vi "HFRR ADV v09.vi"() -> ()   [LabVIEW 2025] (continued)
        n1021 = call-poly "VISA Configure Serial Port"("VISA resource name"=refnum<visa-resource-name> "ASRL1::INSTR" ("COM PORT"), "timeout (10sec)"=u32 10, "baud rate (9600)"=u32 57600, "data bits (8)"=u16 8, "stop bits (10: 1 bit)"=w1236) -> ("VISA resource name out"=w1222:refnum<visa-resource-name>, "error out"=w1231:errorcluster)  [unwired: 9 in]
        n1022 = VISA Read(VISA resource name=w1222, byte count=u32 2 ("byte count (0)")) -> (read buffer=w1230:string)  [unwired: 1 in, 3 out]
        n1023 = String Subset(string=w1230, offset (0)=0, length (rest)=2 ("length (rest)")) -> (substring=w1229:string)
        n1024 = Match Pattern(string=w1229, regular expression="<>") -> (offset past match=w1226:i32)  [unwired: 1 in, 3 out]
        n1025 = Greater Or Equal?(x=w1226, y=0) -> (x >= y?=w1221:bool)
        n1026 = case shown="True" w1221 {
          tunnel: w1222 -> [_ w1240]
          tunnel: w1231 -> [_ w1239]
          frame False {
          }
          frame True {
            n1027 = VISA Read(VISA resource name=w1240, byte count=u32 32 ("byte count (0)"), error in (no error)=w1239) -> (read buffer=w1238:string)  [unwired: 3 out]
            n1028 = String Subset(string=w1238, offset (0)=0, length (rest)=8 ("length (rest)")) -> (substring=w1242:string)
            n1029 = String Subset(string=w1238, offset (0)=8, length (rest)=8 ("length (rest)")) -> (substring=w1243:string)
            n1030 = Decimal String To Number(string=w1243) -> (number=w1250:i32)  [unwired: 2 in, 1 out]
            n1031 = Decimal String To Number(string=w1242) -> (number=w1246:i32)  [unwired: 2 in, 1 out]
            n1032 = Divide(x=w1250, y=10000) -> ()  [unwired: 1 out]
            n1033 = Divide(x=w1246, y=1000000) -> ()  [unwired: 1 out]
          }
        }
        n1034 = local read "Quit"() -> (w1219:bool)
      }
    }
    frame Enabled {
    }
  }
  n1035 = local write "Err Count"(0 ("Err Count")) -> ()
  n1036 = local write "FRICVALZ"(0.0 ("FRICVALZ")) -> ()
  n1037 = Tick Count (ms)() -> (millisecond timer value=w44:u32)
  n1038 = while {
    shift-right: [w1269] -> w48
    shift-left: _ -> [w1258]
    shift-right: [w1268] -> w47
    shift-left: errorcluster {"status"=TRUE, "code"=0, "source"="Init"} ("error IO") -> [w1260]
    shift-right: [w1266] -> _
    shift-left: w44 -> [w1267]
    tunnel: [w1252] -> w35
    tunnel: [w1265] -> _
    i -> [w1265]
    stop <- w1252 stop-if-true
    n1039 = local read "Com Port 1"() -> (w1259:refnum<visa-resource-name>)
    n1040 = local read "Port 1a"() -> (w1261:bool)
    n1041 = local read "Port 3"() -> (w1262:bool)
    n1042 = Not Equal?(x=w1259, y=w1258) -> (x != y?=w1257:bool)
    n1043 = Or(x=w1262, y=w1261) -> (x .or. y?=w1264:bool)
    n1044 = Unbundle(w1260) -> ("status"=→"Port 3":bool)  [unwired: 2 out]
    n1045 = flat-sequence {
      tunnel: [w1272] -> w1256
      tunnel: w1260 -> [w1272]
      frame #0 {
        n1046 = Wait (ms)(milliseconds to wait=u32 200) -> ()  [unwired: 1 out]
      }
    }
    n1047 = case shown="False" w1264 {
      frame False {
        w1274 = FALSE ("Visible")
        n1048 = property on="Port 1a" class="Bool (strict)"("Visible"=w1274) -> ()  [unwired: 2 in, 2 out]
        n1049 = property on="Port 3" class="Bool (strict)"("Visible"=w1274) -> ()  [unwired: 2 in, 2 out]
      }
      frame True {
        w1275 = TRUE ("Visible")
        n1050 = property on="Port 1a" class="Bool (strict)"("Visible"=w1275) -> ()  [unwired: 2 in, 2 out]
        n1051 = property on="Port 3" class="Bool (strict)"("Visible"=w1275) -> ()  [unwired: 2 in, 2 out]
      }
    }
    n1052 = local read "Re-Initialise"() -> (w1253:bool)
    n1053 = Or(x=w1257, y=w1253) -> (x .or. y?=w1254:bool)
    n1054 = case shown="True" w1254 {
      tunnel: [w1270 errorcluster {"status"=TRUE, "code"=0, "source"="Init"} ("error out")] -> w1255
      tunnel: w1256 -> [w1270 _]
      frame False {
      }
      frame True {
      }
    }
    n1055 = case shown="No Error" w1255 {
      selector: w1255 -> [w1276 w1602]
      tunnel: [w1281 w1607] -> w1269
      tunnel: [w1280 w1599] -> w1268
      tunnel: w1258 -> [w1279 w1605]
      tunnel: w1267 -> [w1278 w1604]
      tunnel: [w1277 w1604] -> w1266
      frame No Error {
        n1056 = stacked-sequence {
          tunnel: [w1291 _ _ _ _ _] -> w1281
          tunnel: [w1290 _ _ _ _ _] -> w1280
          tunnel: w1279 -> [w1286 _ _ _ _ _]
          tunnel: w1276 -> [w1285 _ _ _ _ _]
          tunnel: w1278 -> [_ w1399 _ _ _ _]
          tunnel: [_ w1398 _ _ _ _] -> w1277
          tunnel: [_ w1370 _ _ _ _] -> _
          frame #0 {
            n1057 = property class="Instr"(reference=w1286, error in=w1285) -> (reference out=w1288:refnum<visa-resource-name>, error out=w1289:errorcluster, "Serial Settings:Number of Bytes at Serial Port"=w1282:u32)
            "Sps 3" <- w1282
            "Port 1" <- w1282
            n1058 = Greater?(x=w1282, y=u32 5) -> (0:w1284:bool)
            n1059 = case shown="True" w1284 {
              tunnel: w1288 -> [w1293 w1314]
              tunnel: w1289 -> [w1292 w1315]
              tunnel: [w1292 w1317] -> w1290
              tunnel: [w1293 w1316] -> w1291
              frame False {
              }
              frame True {
                # "Out as Volts"
                n1060 = local read "Residual Uno"() -> (w1308:string)
                n1061 = while {
                  tunnel: [w1354] -> w1317
                  tunnel: [w1353] -> w1316
                  tunnel: w1315 -> [w1352]
                  tunnel: w1314 -> [w1351]
                  tunnel: [w1348] -> _
                  shift-right: [w1344] -> w1296
                  shift-left: w1308 -> [w1346]
                  i -> [w1348]
                  stop <- w1349 stop-if-true
                  n1062 = property class="Instr"(reference=w1351, error in=w1352) -> (reference out=w1356:refnum<visa-resource-name>, error out=w1355:errorcluster, "Serial Settings:Number of Bytes at Serial Port"=w1347:u32)
                  n1063 = VISA Read(VISA resource name=w1356, byte count=w1347, error in (no error)=w1355) -> (VISA resource name out=w1353:refnum<visa-resource-name>, read buffer=w1345:string, error out=w1354:errorcluster)  [unwired: 1 out]
                  n1064 = Greater?(x=w1347, y=u32 30) -> (0:w1349:bool)
                  n1065 = Concatenate Strings(w1346, w1345) -> (w1344:string)
                }
                "UnoRead" <- w1296
                n1066 = while {
                  shift-right: [w1330] -> w1307
                  shift-left: w1296 -> [w1336]
                  tunnel: [w1329] -> w1303 mode=indexing
                  tunnel: [w1331] -> _
                  i -> [w1331]
                  stop <- w1333 stop-if-true
                  n1067 = Match Pattern(string=w1336, regular expression="*") -> (after substring=w1334:string)  [unwired: 1 in, 3 out]
                  n1068 = Match Pattern(string=w1334, regular expression="&") -> (before substring=w1329:string, after substring=w1330:string, offset past match=w1332:i32)  [unwired: 1 in, 1 out]
                  n1069 = Less Than 0?(x=w1332) -> (x < 0?=w1333:bool)
                }
                n1070 = local write "Residual Uno"(w1307) -> ()
                n1071 = Array Size(array=w1303) -> (size(s)=w1304:i32)
                n1072 = Decrement(x=w1304) -> (x-1=w1306:i32)
                n1073 = Delete From Array(array=w1303, length=1, index=w1306) -> (array with subset deleted=w1301:string[])  [unwired: 1 out]
                n1074 = Array Size(array=w1301) -> (size(s)=w1300:i32)
                n1075 = Decrement(x=w1300) -> (x-1=w1299:i32)
                n1076 = while {
                  tunnel: [w1328] -> w1312 mode=indexing
                  tunnel: [w1327] -> w1311 mode=indexing
                  tunnel: w1301 -> [w1321] mode=indexing
                  tunnel: w1299 -> [w1320]
                  tunnel: [w1318] -> _
                  i -> [w1318]
                  stop <- w1319 stop-if-true
                  w1322 = 0 ("length (rest)")
                  w1324 = ";" ("regular expression")
                  n1077 = Less Or Equal?(x=w1320, y=w1318) -> (x <= y?=w1319:bool)
                  n1078 = Match Pattern(string=w1321, regular expression=w1324) -> (before substring=w1326:string, after substring=w1325:string)  [unwired: 1 in, 2 out]
                  n1079 = Decimal String To Number(string=w1326, default (0L)=w1322) -> (number=w1328:i32)  [unwired: 1 in, 1 out]
                  n1080 = Match Pattern(string=w1325, regular expression=w1324) -> (before substring=w1323:string)  [unwired: 1 in, 3 out]
                  n1081 = Decimal String To Number(string=w1323, default (0L)=w1322) -> (number=w1327:i32)  [unwired: 1 in, 1 out]
                }
                n1082 = case shown="0, Default" "ADC Res" {
                  tunnel: [w1339 w1341] -> w1295
                  frame 0, Default {
                    n1083 = Divide(x=65535 ("length (rest)"), y=2 ("length (rest)")) -> (x/y=w1339:dbl)
                  }
                  frame 1 {
                    n1084 = Divide(x=16777216 ("length (rest)"), y=2 ("length (rest)")) -> (x/y=w1341:dbl)
                  }
                }
                n1085 = Bundle(w1312, w1311) -> (w1302:cluster{i32[], i32[]})  [unwired: 1 in]
                n1086 = Divide(x=w1302, y=w1295) -> (x/y=w1313:cluster{dbl[], dbl[]})
                n1087 = Multiply(x=w1313, y=sgl 5.03 ("Numeric")) -> (x*y=w1310:cluster{dbl[], dbl[]})
                n1088 = Unbundle(w1310) -> (→"Ch1":dbl[], →"Ch0":dbl[])
              }
            }
            n1089 = Not(x=w1284) -> (.not. x?=→"Port 1a":bool)
          }
          frame #1 {
            n1090 = local read "zOff 2"() -> (w1391:dbl)
            n1091 = local read "Ch1"() -> (w1381:dbl[])
            n1092 = case shown="True" "Zero 2" {
              tunnel: w1381 -> [_ w1411]
              frame False {
              }
              frame True {
                n1093 = call-poly <vilib>:"Mean.vi"("X"=w1411) -> ("mean"=→"zOff 2":dbl)  [unwired: 1 out]
                n1094 = local write "Zero 2"(FALSE ("Zero")) -> ()
              }
            }
            n1095 = Subtract(x=w1381, y=w1391) -> (x-y=w1387:dbl[])
            n1096 = call-poly <vilib>:"Mean.vi"("X"=w1381) -> ("mean"=w1382:dbl)  [unwired: 1 out]
            "Slide 3" <- w1382
            n1097 = Multiply(x=w1387, y=1.0 ("PG Oth")) -> (x*y=w1373:dbl[])
            n1098 = local read "FF buffer"() -> (w1378:dbl[])
            n1099 = Divide(x=w1373, y=1) -> (x/y=w1372:dbl[])
            "Fric Val" <- w1372
            n1100 = call <vilib>:"Mean PtByPt.vi"("x"=w1382, "sample length"=10, "initialize"="Reset 2") -> ("mean"=→"Mean Pos Fil 2":dbl)  [unwired: 1 in, 1 out]
            n1101 = Array Size(array=w1378) -> (size(s)=w1380:i32)
            n1102 = call-poly <vilib>:"Mean.vi"("X"=w1372) -> ("mean"=w1386:dbl)  [unwired: 1 out]
            n1103 = Insert Into Array(array=w1378, index=w1380, new element=w1372) -> (w1375:dbl[])
            n1104 = Array Size(array=w1375) -> (size(s)=w1374:i32)
            n1105 = case shown="True" "DC corr 2" {
              tunnel: w1372 -> [w1414 w1417]
              tunnel: [w1414 w1416] -> w1379
              tunnel: w1386 -> [_ w1415]
              frame False {
              }
              frame True {
                n1106 = Subtract(x=w1417, y=w1415) -> (x-y=w1416:dbl[])
              }
            }
            n1107 = Tick Count (ms)() -> (millisecond timer value=w1398:u32)
            n1108 = Greater?(x=w1374, y=1000) -> (0:w1376:bool)
            n1109 = Subtract(x=w1398, y=w1399) -> (x-y=w1397:u32)
            n1110 = case shown="True" w1376 {
              tunnel: [w1404 w1407] -> w1363
              tunnel: w1375 -> [w1404 w1410]
              tunnel: w1374 -> [_ w1409]
              frame False {
              }
              frame True {
                n1111 = Subtract(x=w1409, y=1000) -> (x-y=w1405:i32)
                n1112 = Delete From Array(array=w1410, length=w1405, index=0) -> (array with subset deleted=w1407:dbl[])  [unwired: 1 out]
              }
            }
            n1113 = Divide(x=w1397, y=u32 1000 ("x")) -> (x/y=w1395:dbl)
            n1114 = Array Size(array=w1379) -> (size(s)=w1394:i32)
            n1115 = Divide(x=w1394, y=w1395) -> (x/y=w1390:dbl)
            "Sps 2" <- w1390
            n1116 = Reciprocal(x=w1390) -> (1/x=w1388:dbl)
            "dt" <- w1388
            n1117 = local read "FRIC. FORCE :"() -> (w1360:dbl)
            n1118 = local write "FF buffer"(w1363) -> ()
            n1119 = Negate(x=w1363) -> (-x=w1362:dbl[])
            n1120 = call "Elapsed Time5"("Time Target (s)"="check time s", "Reset"="Reset 3") -> ("Time has Elapsed"=w1365:bool)  [unwired: 10 in, 7 out]
            n1121 = Array Max & Min(array=w1362) -> (max value=w1370:dbl)  [unwired: 3 out]
            n1122 = Bundle By Name("Y"=w1379, "dt"=w1388, "t0"=timestamp(0 s since 1904-01-01)) -> (w1358:waveform(dbl))  [unwired: 1 in]
            n1123 = Multiply(x=w1360, y=21.1986) -> (x*y=w1359:dbl)
            n1124 = Greater Or Equal?(x=w1370, y="Threshold value") -> (x >= y?=w1366:bool)
            n1125 = Multiply(x=w1359, y=w1358) -> (x*y=→"FF_Wfm":waveform(dbl))
            n1126 = And(x=w1366, y=w1365) -> (x .and. y?=w1364:bool)
            n1127 = case shown="True" w1364 {
              frame False {
                n1128 = local write "Reset 3"(FALSE ("Reset 3")) -> ()
              }
              frame True {
                n1129 = local write "Reset 3"(TRUE ("Reset 3")) -> ()
                n1130 = local write "save dpt"(TRUE ("save dpt")) -> ()
              }
            }
          }
          frame #2 {
            n1131 = local read "FF buffer"() -> (w1424:dbl[])
            n1132 = Array Max & Min(array=w1424) -> (max value=w1419:dbl, min value=w1420:dbl)  [unwired: 2 out]
            n1133 = Subtract(x=w1419, y=w1420) -> (x-y=w1421:dbl)
            n1134 = Multiply(x=1.0 ("y 2"), y="Threshold") -> ()  [unwired: 1 out]
            n1135 = Greater?(x=w1421, y="Threshold") -> (0:w1418:bool)
            n1136 = case shown="True" w1418 {
              tunnel: w1424 -> [_ w1431]
              tunnel: [_ w1429] -> _
              frame False {
              }
              frame True {
                w1430 = 1.0 ("y")
                n1137 = Delete From Array(array=w1431, length=100, index=0) -> (deleted portion=w1436:dbl[])  [unwired: 1 out]
                n1138 = call-poly <vilib>:"Mean.vi"("X"=w1436) -> ("mean"=w1435:dbl)  [unwired: 1 out]
                n1139 = Subtract(x=w1431, y=w1435) -> (x-y=w1434:dbl[])
                n1140 = Multiply(x=w1430, y=w1430) -> (x*y=w1432:dbl)
                n1141 = Multiply(x=w1434, y=w1432) -> (x*y=w1433:dbl[])
                "FF cal val" <- w1433
                n1142 = Array Size(array=w1433) -> (size(s)=w1427:i32)
                n1143 = Array Max & Min(array=w1433) -> (max value=w1426:dbl, min value=w1425:dbl)  [unwired: 2 out]
                n1144 = property on="FF Calibration g" class="WFGraph (strict)"("X Scale.Range:Minimum"=0.0 ("y"), "X Scale.Range:Maximum"=w1427, "Y Scale.Range:Minimum"=w1426, "Y Scale.Range:Maximum"=w1425) -> ()  [unwired: 2 in, 2 out]
                n1145 = local read "FRIC. FORCE :"() -> (w1429:dbl)
              }
            }
          }
          frame #3 {
            # "5"
            n1146 = local read "DISPLACEMENT :"() -> (w1524:dbl)
            n1147 = Multiply(x=w1524, y=1.0) -> (x*y=w1441:dbl)
            n1148 = local read "zOff 3"() -> (w1527:dbl)
            n1149 = local read "Ch0"() -> (w1454:dbl[])
            n1150 = case shown="True" "Zero 3" {
              tunnel: w1454 -> [_ w1542]
              frame False {
              }
              frame True {
                n1151 = call-poly <vilib>:"Mean.vi"("X"=w1542) -> ("mean"=→"zOff 3":dbl)  [unwired: 1 out]
                n1152 = local write "Zero 3"(FALSE ("Zero")) -> ()
              }
            }
            n1153 = Add(x=w1454, y="Offset") -> (x+y=w1453:dbl[])
            n1154 = Multiply(x=w1441, y="DISPLACEMENT : 2") -> (x*y=w1508:dbl)
            n1155 = Subtract(x=w1454, y=w1527) -> (x-y=w1511:dbl[])
            n1156 = Multiply(x=w1511, y=w1508) -> (x*y=w1510:dbl[])
            n1157 = Multiply(x=w1511, y=w1441) -> (x*y=w1523:dbl[])
            "ABS DP" <- w1523
            n1158 = local read "Standard Slip Gauge (mm)"() -> (w1509:dbl)
            n1159 = call-poly <vilib>:"Mean.vi"("X"=w1510) -> ("mean"=w1440:dbl)  [unwired: 1 out]
            "Disp (mm)" <- w1440
            "software msrnt" <- w1440
            n1160 = Multiply(x=w1453, y="Gain") -> (x*y=w1448:dbl[])
            "Voltage LVDT Acq" <- w1448
            "gLVDTraw" <- w1448
            n1161 = call-poly <vilib>:"Mean.vi"("X"=w1523) -> ("mean"=w1513:dbl)  [unwired: 1 out]
            n1162 = case shown="True" "DC correction" {
              tunnel: w1523 -> [w1545 w1548]
              tunnel: [w1545 w1547] -> w1460
              tunnel: w1513 -> [_ w1546]
              frame False {
              }
              frame True {
                n1163 = Subtract(x=w1548, y=w1546) -> (x-y=w1547:dbl[])
              }
            }
            n1164 = Divide(x=w1440, y=w1509) -> (x/y=w1507:dbl)
            n1165 = call-poly <vilib>:"Mean.vi"("X"=w1448) -> ("mean"=w1447:dbl)  [unwired: 1 out]
            n1166 = Array Max & Min(array=w1448) -> (max value=w1452:dbl, min value=w1451:dbl)  [unwired: 2 out]
            n1167 = Multiply(x=w1507, y=w1508) -> (x*y=→"DISPLACEMENT : 3":dbl)
            n1168 = Subtract(x=w1452, y=w1451) -> (x-y=→"Pk-Pk":dbl)
            n1169 = local read "dt"() -> (w1526:dbl)
            n1170 = Threshold 1D Array(2:0.0 ("threshold y"), 3:w1460) -> (0:w1477:dbl)  [unwired: 1 in]
            n1171 = Bundle By Name("Y"=w1460, "dt"=w1526, "t0"=timestamp(0 s since 1904-01-01)) -> (w1515:waveform(dbl))  [unwired: 1 in]
            n1172 = local read "FF_Wfm"() -> (w1514:waveform(dbl))
            n1173 = Equal To 0?(x=w1477) -> (x = 0?=w1478:bool)
            n1174 = case shown="True" w1478 {
              tunnel: w1460 -> [_ w1536]
              tunnel: [w1532 w1533] -> w1473
              tunnel: w1477 -> [w1532 _]
              frame False {
              }
              frame True {
                n1175 = Threshold 1D Array(1:20 ("start index (0)"), 2:0.0 ("threshold y"), 3:w1536) -> (0:w1533:dbl)
              }
            }
            n1176 = call-poly <vilib>:"Extract Single Tone Information.vi"("time signal in"=w1515) -> ("detected amplitude"=w1449:dbl, "detected frequency"=→"Freq":dbl)  [unwired: 5 in, 4 out]
            n1177 = Build Array(w1515, w1514) -> (w1496:waveform(dbl)[])
            "Waveform Graph 2" <- w1496
            n1178 = Subtract(x=w1447, y="LvdtOff") -> (x-y=w1446:dbl)
            n1179 = Subtract(x=w1446, y=w1449) -> (x-y=w1458:dbl)
            n1180 = Add(x=w1449, y=w1446) -> (x+y=w1457:dbl)
            n1181 = Index Array(array=w1496) -> (element #1=w1497:waveform(dbl), element #2=w1499:waveform(dbl))  [unwired: 2 in]
            n1182 = Multiply(x=w1449, y=2.0) -> (x*y=w1516:dbl)
            "Stroke" <- w1516
            "Mean(RAW) Stroke" <- w1516
            n1183 = Bundle(w1446, w1458, w1457) -> (→"Slide 8":cluster{dbl, dbl, dbl})  [unwired: 1 in]
            n1184 = Unbundle By Name(w1497) -> ("Y"=w1470:dbl[])
            n1185 = Split 1D Array(array=w1460, index=w1473) -> (second subarray=w1474:dbl[])  [unwired: 1 out]
            n1186 = In Range and Coerce(upper limit=1.5, x=w1516, lower limit=0.5) -> (In Range?=w1520:bool)  [unwired: 1 out]
            n1187 = Split 1D Array(array=w1470, index="Window") -> (second subarray=w1488:dbl[])  [unwired: 1 out]
            n1188 = Unbundle By Name(w1499) -> ("Y"=w1471:dbl[])
            n1189 = Threshold 1D Array(1:180 ("start index (0)"), 2:0.0 ("threshold y"), 3:w1474) -> (0:w1472:dbl)
            n1190 = local read "Test \nStatus"() -> (w1517:bool)
            n1191 = Split 1D Array(array=w1471, index=w1473) -> (second subarray=w1468:dbl[])  [unwired: 1 out]
            n1192 = Not(x=w1520) -> (.not. x?=w1519:bool)
            n1193 = call-poly <vilib>:"RMS.vi"("X"=w1488) -> ("rms value"=w1444:dbl)  [unwired: 1 out]
            "Current (A)" <- w1444
            n1194 = Array Max & Min(array=w1488) -> (max value=w1502:dbl, min value=w1503:dbl)  [unwired: 2 out]
            n1195 = Array Max & Min(array=w1471) -> (max value=w1500:dbl, min value=w1501:dbl)  [unwired: 2 out]
            n1196 = Subtract(x=w1502, y=w1503) -> (x-y=w1504:dbl)
            n1197 = Subtract(x=w1500, y=w1501) -> (x-y=w1505:dbl)
            n1198 = And(x=w1519, y=w1517) -> (x .and. y?=w1518:bool)
            n1199 = Split 1D Array(array=w1474, index=w1472) -> (first subarray=w1467:dbl[])  [unwired: 1 out]
            n1200 = Split 1D Array(array=w1468, index=w1472) -> (first subarray=w1465:dbl[])  [unwired: 1 out]
            n1201 = case shown="True" w1518 {
              tunnel: [i32[] [] w1538] -> _
              frame False {
              }
              frame True {
                n1202 = local read "UnoRead"() -> (w1540:string)
                n1203 = local read "Array"() -> (w1541:string[])
                n1204 = Build Array (concatenate)(w1541, w1540) -> (w1539:string[])
                "Array" <- w1539
                n1205 = String Length(string=w1539) -> (length=w1538:i32[])
              }
            }
            n1206 = local read "G_val"() -> (w1490:dbl)
            n1207 = Divide(x=w1505, y=w1504) -> (x/y=w1493:dbl)
            n1208 = call-poly <vilib>:"RMS.vi"("X"=w1465) -> ("rms value"=w1489:dbl)  [unwired: 1 out]
            n1209 = call-poly <vilib>:"Hanning Window.vi"("X"=w1467) -> ("Windowed X"=w1466:dbl[])  [unwired: 1 out]
            n1210 = call-poly <vilib>:"Hanning Window.vi"("X"=w1465) -> ("Windowed X"=w1464:dbl[])  [unwired: 1 out]
            n1211 = local read "Constant (G)"() -> (w1482:dbl)
            n1212 = Divide(x=w1489, y=w1444) -> (x/y=w1483:dbl)
            n1213 = Build Array(w1466, w1464) -> (→"Waveform Graph 4":dbl[][])
            n1214 = Multiply(x=w1493, y=0.2) -> (x*y=w1495:dbl)
            n1215 = Multiply(x=0.8 ("y"), y=w1490) -> (x*y=w1494:dbl)
            n1216 = Add(x=w1495, y=w1494) -> (x+y=w1462:dbl)
            n1217 = Multiply(x=w1483, y=0.2) -> (x*y=w1484:dbl)
            n1218 = Multiply(x=0.8 ("y"), y=w1482) -> (x*y=w1485:dbl)
            n1219 = Add(x=w1484, y=w1485) -> (x+y=w1481:dbl)
            "Constant (G)" <- w1481
            n1220 = Not A Number/Path/Refnum?(number/path/refnum=w1462) -> (NaN/Path/Refnum?=w1461:bool)
            n1221 = Select(t=0.0, s=w1461, f=w1462) -> (s? t:f=w1442:dbl)
            "G_val" <- w1442
            n1222 = Multiply(x=w1444, y=w1442) -> (x*y=→"Friction Force (N)":dbl)
            n1223 = Bundle(w1481, "t"=w1442) -> (→"pk-pk":cluster{dbl, "t":dbl})  [unwired: 1 in]
          }
          frame #4 {
            # "C:\\WinDucom\\data\\"
            # "?C:\\LAB-IQ-NXT\\data"
            n1224 = case shown="True" "save dpt" {
              frame False {
              }
              frame True {
                n1225 = local write "save dpt"(FALSE ("Hold 3")) -> ()
                n1226 = local read "file count"() -> (w1552:i32)
                n1227 = Number To Decimal String(number=w1552) -> (decimal integer string=w1558:string)  [unwired: 1 in]
                n1228 = Add(x=1, y=w1552) -> (x+y=w1553:i32)
                n1229 = local write "file count"(w1553) -> ()
                n1230 = local read "FILE 2"() -> (w1557:string)
                n1231 = Concatenate Strings(w1557, w1558) -> (w1550:string)
                n1232 = Concatenate Strings("C:\\LAB-IQ\\data" ("Substring"), w1550) -> (w1565:string)
                n1233 = local read "FF buffer"() -> (w1560:dbl[])
                n1234 = local read "ABS DP"() -> (w1559:dbl[])
                n1235 = Concatenate Strings(w1565, ".dpf" ("Substring")) -> (w1563:string)
                n1236 = Build Array(w1560, w1559) -> (w1555:dbl[][])
                n1237 = Concatenate Strings("FF ( V ); DP( mincron ) " ("character string"), "\r") -> (w1569:string)
                n1238 = String To Path(string=w1563) -> (path=w1561:path)
                n1239 = Transpose 2D Array(2D array=w1555) -> (transposed array=w1554:dbl[][])
                n1240 = call <vilib>:"Write Characters To File.vi"("append to file? (new file:F)"=FALSE, "character string"=w1569, "file path (dialog if empty)"=w1561) -> ("new file path (Not A Path if cancelled)"=w1566:path)  [unwired: 2 in]
                n1241 = Array To Spreadsheet String(delimiter (Tab)=";", array=w1554, 3:"" ("format string")) -> (spreadsheet string=w1556:string)
                "String 9" <- w1556
                n1242 = call <vilib>:"Write Characters To File.vi"("append to file? (new file:F)"=TRUE, "character string"=w1556, "file path (dialog if empty)"=w1566) -> ()  [unwired: 2 in, 1 out]
              }
            }
          }
          frame #5 {
            n1243 = case shown="True" "Hold 4" {
              frame False {
              }
              frame True {
                n1244 = File Dialog(6:"*.dpf" ("pattern"), 11:path "C:/LAB-IQ" ("start path")) -> (0:w1576:errorcluster, 3:w1591:path)  [unwired: 5 in, 2 out]
                n1245 = Unbundle(w1576) -> ()  [unwired: 3 out]
                n1246 = call <vilib>:"Read Characters From File.vi"("file path (dialog if empty)"=w1591) -> ("character string"=w1581:string)  [unwired: 5 in, 3 out]
                n1247 = Spreadsheet String To Array(delimiter (Tab)=";", format string="%S", spreadsheet string=w1581, array type (2D Dbl)=string[][] []) -> (array=w1585:string[][])
                n1248 = for {
                  tunnel: w1585 -> [w1595] mode=indexing
                  tunnel: [w1594] -> w1586 mode=indexing
                  n1249 = for {
                    tunnel: w1595 -> [w1597] mode=indexing
                    tunnel: [w1596] -> w1594 mode=indexing
                    n1250 = call <vilib>:"Trim Whitespace.vi"("string"=w1597) -> ("trimmed string"=w1596:string)  [unwired: 1 in]
                  }
                }
                n1251 = Fract/Exp String To Number(string=w1586) -> (number=w1588:dbl[][])  [unwired: 3 in, 1 out]
                n1252 = Array Subset(array=w1588, index (row)=1 ("index (col)")) -> (w1590:dbl[][])  [unwired: 3 in]
                n1253 = Index Array(array=w1590, index (col) #1=0 ("disabled index (col)"), index (col) #2=1 ("disabled index (col)")) -> (element #1=w1579:dbl[], element #2=w1578:dbl[])  [unwired: 2 in]
                n1254 = Build Array(w1579, w1578) -> (→"Waveform Graph":dbl[][])
              }
            }
          }
        }
      }
      frame Error {
        w1613 = u16 0 items=["None", "XON/XOFF", "RTS/CTS", "XON/XOFF & RTS/CTS", "DTR/DSR", "XON/XOFF & DTR/DSR"] ("flow control (0:none)  2")
        w1611 = u16 10 items=["1.0"=10, "1.5"=15, "2.0"=20] ("stop bits 2")
        w1609 = u16 0 items=["None", "Odd", "Even", "Mark", "Space"] ("parity 2")
        w1610 = u32 10000  # timeout (10sec)
        n1255 = VISA Close(VISA resource name=w1605, error in (no error)=w1602) -> (error out=w1606:errorcluster)
        n1256 = local write "Sps 3"(0.0 ("Sps 4")) -> ()
        n1257 = call <vilib>:"Clear Errors.vi"("error in (no error)"=w1606) -> ("error out"=w1603:errorcluster)  [unwired: 5 in, 1 out]
        n1258 = local read "Com Port 1"() -> (w1598:refnum<visa-resource-name>)
        n1259 = call-poly "VISA Configure Serial Port"("VISA resource name"=w1598, "timeout (10sec)"=w1610, "baud rate (9600)"=u32 250000 ("baud rate  2"), "data bits (8)"=u16 8 ("data bits  2"), "parity (0:none)"=w1609, "error in (no error)"=w1603, "stop bits (10: 1 bit)"=w1611, "flow control (0:none)"=w1613) -> ("VISA resource name out"=w1614:refnum<visa-resource-name>, "error out"=w1615:errorcluster)  [unwired: 6 in]
        n1260 = flat-sequence {
          tunnel: w1614 -> [w1617]
          tunnel: w1615 -> [w1616]
          tunnel: [w1617] -> w1607
          tunnel: [w1616] -> w1599
          frame #0 {
            n1261 = Wait (ms)(milliseconds to wait=u32 50) -> ()  [unwired: 1 out]
          }
        }
        "Residual Uno" <- ""
        "Port 1 Error" <- w1599
      }
    }
    n1262 = local read "Quit"() -> (w1252:bool)
    "Error Uno" <- w1260
  }
  n1263 = while {
    shift-right: [w1634] -> w29
    shift-left: _ -> [w1625]
    shift-right: [w1633] -> w28
    shift-left: errorcluster {"status"=FALSE, "code"=0, "source"="Init"} ("error out") -> [w1627]
    tunnel: [w1619] -> w34
    tunnel: [w1632] -> _
    i -> [w1632]
    stop <- w1619 stop-if-true
    n1264 = local read "Com Port 2"() -> (w1626:refnum<visa-resource-name>)
    n1265 = local read "Port 2a"() -> (w1628:bool)
    n1266 = local read "Port 4"() -> (w1629:bool)
    n1267 = Not Equal?(x=w1626, y=w1625) -> (x != y?=w1624:bool)
    n1268 = Or(x=w1629, y=w1628) -> (x .or. y?=w1631:bool)
    n1269 = Unbundle(w1627) -> ("status"=→"Port 4":bool)  [unwired: 2 out]
    n1270 = flat-sequence {
      tunnel: w1627 -> [w1638]
      tunnel: [w1638] -> w1623
      frame #0 {
        n1271 = Wait (ms)(milliseconds to wait=u32 50) -> ()  [unwired: 1 out]
      }
    }
    n1272 = local read "Re-Initialise"() -> (w1620:bool)
    n1273 = case shown="True" w1631 {
      frame False {
        w1639 = FALSE ("Visible")
        n1274 = property on="Port 2a" class="Bool (strict)"("Visible"=w1639) -> ()  [unwired: 2 in, 2 out]
        n1275 = property on="Port 4" class="Bool (strict)"("Visible"=w1639) -> ()  [unwired: 2 in, 2 out]
      }
      frame True {
        w1640 = TRUE ("Visible")
        n1276 = property on="Port 2a" class="Bool (strict)"("Visible"=w1640) -> ()  [unwired: 2 in, 2 out]
        n1277 = property on="Port 4" class="Bool (strict)"("Visible"=w1640) -> ()  [unwired: 2 in, 2 out]
      }
    }
    n1278 = Or(x=w1624, y=w1620) -> (x .or. y?=w1621:bool)
    n1279 = case shown="True" w1621 {
      tunnel: [w1635 errorcluster {"status"=TRUE, "code"=0, "source"="Init"} ("error out")] -> w1622
      tunnel: w1623 -> [w1635 _]
      frame False {
      }
      frame True {
      }
    }
    n1280 = case shown="Error" w1622 {
      selector: w1622 -> [w1641 w1795]
      tunnel: [w1643 w1800] -> w1634
      tunnel: [w1642 w1793] -> w1633
      tunnel: w1625 -> [w1645 w1798]
      tunnel: [w1644 _] -> _
      frame No Error {
        n1281 = stacked-sequence {
          tunnel: w1645 -> [w1669 _]
          tunnel: w1641 -> [w1668 _]
          tunnel: [w1655 _] -> w1644
          tunnel: [w1654 _] -> w1643
          tunnel: [w1653 _] -> w1642
          frame #0 {
            n1282 = property class="Instr"(reference=w1669, error in=w1668) -> (reference out=w1652:refnum<visa-resource-name>, error out=w1667:errorcluster, "Serial Settings:Number of Bytes at Serial Port"=w1648:u32)
            "Port 2" <- w1648
            n1283 = Greater?(x=w1648, y=u32 23) -> (0:w1650:bool)
            n1284 = Not(x=w1650) -> ()  [unwired: 1 out]
            n1285 = case shown="True" w1650 {
              tunnel: w1652 -> [w1684 w1709]
              tunnel: w1667 -> [w1683 w1710]
              tunnel: [w1683 w1712] -> w1663
              tunnel: [w1684 w1711] -> w1664
              frame False {
              }
              frame True {
                # "Out as Volts"
                n1286 = local read "Residual Due"() -> (w1708:string)
                n1287 = while {
                  tunnel: [w1752] -> w1712
                  tunnel: [w1751] -> w1711
                  tunnel: w1710 -> [w1750]
                  tunnel: w1709 -> [w1749]
                  tunnel: [w1746] -> _
                  shift-right: [w1744] -> w1707
                  shift-left: w1708 -> [w1743]
                  i -> [w1746]
                  stop <- w1747 stop-if-true
                  n1288 = property class="Instr"(reference=w1749, error in=w1750) -> (reference out=w1754:refnum<visa-resource-name>, error out=w1753:errorcluster, "Serial Settings:Number of Bytes at Serial Port"=w1745:u32)
                  n1289 = VISA Read(VISA resource name=w1754, byte count=w1745, error in (no error)=w1753) -> (VISA resource name out=w1751:refnum<visa-resource-name>, read buffer=w1742:string, error out=w1752:errorcluster)  [unwired: 1 out]
                  n1290 = Greater?(x=w1745, y=u32 8) -> (0:w1747:bool)
                  n1291 = Concatenate Strings(w1743, w1742) -> (w1744:string)
                }
                n1292 = while {
                  shift-right: [w1735] -> w1691
                  shift-left: w1707 -> [w1740]
                  tunnel: [w1734] -> w1703 mode=indexing
                  tunnel: [w1733] -> _
                  i -> [w1733]
                  stop <- w1737 stop-if-true
                  n1293 = Match Pattern(string=w1740, regular expression="*") -> (after substring=w1738:string)  [unwired: 1 in, 3 out]
                  n1294 = Match Pattern(string=w1738, regular expression="&") -> (before substring=w1734:string, after substring=w1735:string, offset past match=w1736:i32)  [unwired: 1 in, 1 out]
                  n1295 = Less Than 0?(x=w1736) -> (x < 0?=w1737:bool)
                }
                n1296 = Array Size(array=w1703) -> (size(s)=w1706:i32)
                n1297 = local write "Residual Due"(w1691) -> ()
                n1298 = Decrement(x=w1706) -> (x-1=w1704:i32)
                n1299 = Delete From Array(array=w1703, length=1, index=w1704) -> (array with subset deleted=w1702:string[])  [unwired: 1 out]
                n1300 = Array Size(array=w1702) -> (size(s)=w1690:i32)
                n1301 = Decrement(x=w1690) -> (x-1=w1689:i32)
                n1302 = while {
                  tunnel: w1702 -> [w1721] mode=indexing
                  tunnel: w1689 -> [w1720]
                  tunnel: [w1718] -> w1697 mode=indexing
                  tunnel: [w1717] -> w1696 mode=indexing
                  tunnel: [w1716] -> w1695 mode=indexing
                  tunnel: [w1715] -> w1694 mode=indexing
                  tunnel: [w1714] -> w1692 mode=indexing
                  tunnel: [w1713] -> _
                  i -> [w1713]
                  stop <- w1719 stop-if-true
                  w1730 = u32 0 ("length (rest)")
                  w1729 = ";" ("regular expression")
                  n1303 = Less Or Equal?(x=w1720, y=w1713) -> (x <= y?=w1719:bool)
                  n1304 = Match Pattern(string=w1721, regular expression=w1729) -> (before substring=w1722:string, after substring=w1723:string)  [unwired: 1 in, 2 out]
                  n1305 = Match Pattern(string=w1723, regular expression=w1729) -> (before substring=w1726:string, after substring=w1724:string)  [unwired: 1 in, 2 out]
                  n1306 = Decimal String To Number(string=w1722, default (0L)=w1730) -> (number=w1718:u32)  [unwired: 1 in, 1 out]
                  n1307 = Decimal String To Number(string=w1726, default (0L)=w1730) -> (number=w1717:u32)  [unwired: 1 in, 1 out]
                  n1308 = Match Pattern(string=w1724, regular expression=w1729) -> (before substring=w1727:string, after substring=w1725:string)  [unwired: 1 in, 2 out]
                  n1309 = Decimal String To Number(string=w1727, default (0L)=w1730) -> (number=w1716:u32)  [unwired: 1 in, 1 out]
                  n1310 = Match Pattern(string=w1725, regular expression=w1729) -> (before substring=w1728:string, after substring=w1732:string)  [unwired: 1 in, 2 out]
                  n1311 = Decimal String To Number(string=w1728, default (0L)=w1730) -> (number=w1715:u32)  [unwired: 1 in, 1 out]
                  n1312 = Decimal String To Number(string=w1732, default (0L)=u8 0 ("length (rest)")) -> (number=w1714:u8)  [unwired: 1 in, 1 out]
                }
                "Din" <- w1692
                n1313 = Bundle(w1697, w1696, w1695, w1694) -> (w1699:cluster{u32[], u32[], u32[], u32[]})  [unwired: 1 in]
                n1314 = Divide(x=w1699, y=4095 ("length (rest)")) -> (x/y=w1701:cluster{dbl[], dbl[], dbl[], dbl[]})
                n1315 = Multiply(x=w1701, y=sgl 3.32 ("Numeric")) -> (x*y=w1693:cluster{dbl[], dbl[], dbl[], dbl[]})
                n1316 = Unbundle(w1693) -> (→"ECR":dbl[], →"Rtemp":dbl[], →"Air temp":dbl[], →"Ch3 2":dbl[])
              }
            }
            n1317 = call "Elapsed Time10"("Time Target (s)"=2.0, "Reset"=w1650, "Auto Reset"=FALSE) -> ("Time has Elapsed"=→"Port 2a":bool)  [unwired: 9 in, 7 out]
            n1318 = local read "Due Com"() -> (w1656:string[])
            n1319 = Array Size(array=w1656) -> (size(s)=w1655:i32)
            n1320 = Delete From Array(array=w1656, length=1, index=0) -> (deleted portion=w1659:string[], array with subset deleted=w1660:string[])
            n1321 = local write "Due Com"(w1660) -> ()
            n1322 = Index Array(array=w1659, index=0) -> (element=w1657:string)
            n1323 = Not Equal?(x=w1657, y="") -> (x != y?=w1665:bool)
            n1324 = case shown="True" w1665 {
              tunnel: w1664 -> [w1671 w1676]
              tunnel: [w1671 w1680] -> w1654
              tunnel: w1663 -> [w1670 w1675]
              tunnel: [w1670 w1678] -> w1653
              tunnel: w1657 -> [_ w1674]
              tunnel: [_ w1677] -> _
              frame False {
                # "DATA  WRITE LOOP"
              }
              frame True {
                n1325 = Concatenate Strings(w1674, "\r\n") -> (w1673:string)
                n1326 = VISA Write(VISA resource name=w1676, write buffer=w1673, error in (no error)=w1675) -> (VISA resource name out=w1680:refnum<visa-resource-name>, return count=w1677:u32, error out=w1679:errorcluster)
                n1327 = flat-sequence {
                  tunnel: w1679 -> [w1681]
                  tunnel: [w1681] -> w1678
                  frame #0 {
                    n1328 = Wait (ms)(milliseconds to wait=u32 5) -> ()  [unwired: 1 out]
                  }
                }
              }
            }
          }
          frame #1 {
            w1763 = 10 ("y")
            w1768 = 10 ("y")
            n1329 = local read "Rtemp"() -> (w1756:dbl[])
            n1330 = local read "ecr buf"() -> (w1757:dbl[])
            n1331 = for {
              tunnel: w1756 -> [w1780] mode=indexing
              shift-right: [w1781] -> w1764
              shift-left: dbl[] [] ("temp buf 2") -> [w1782]
              n1332 = Build Array (concatenate)(w1782, w1780) -> (w1783:dbl[])
              n1333 = Equal To 0?(x=w1780) -> (x = 0?=w1784:bool)
              n1334 = Select(t=w1782, s=w1784, f=w1783) -> (s? t:f=w1781:dbl[])
            }
            n1335 = local read "ECR"() -> (w1755:dbl[])
            n1336 = Insert Into Array(array=w1755, index=0, new element=w1757) -> (w1761:dbl[])
            n1337 = local read "temp buf"() -> (w1765:dbl[])
            n1338 = Array Size(array=w1761) -> (size(s)=w1762:i32)
            n1339 = Greater?(x=w1762, y=w1763) -> (0:w1760:bool)
            n1340 = case shown="True" w1760 {
              tunnel: w1761 -> [w1773 w1779]
              tunnel: w1762 -> [_ w1777]
              tunnel: w1763 -> [_ w1776]
              tunnel: [w1773 w1774] -> w1758
              frame False {
              }
              frame True {
                n1341 = Subtract(x=w1777, y=w1776) -> (x-y=w1775:i32)
                n1342 = Delete From Array(array=w1779, length=w1775, index=0) -> (array with subset deleted=w1774:dbl[])  [unwired: 1 out]
              }
            }
            "ecr buf" <- w1758
            n1343 = Insert Into Array(array=w1764, index=0, new element=w1765) -> (w1770:dbl[])
            n1344 = Array Size(array=w1770) -> (size(s)=w1769:i32)
            n1345 = Greater?(x=w1769, y=w1768) -> (0:w1771:bool)
            n1346 = case shown="True" w1771 {
              tunnel: w1770 -> [w1785 w1791]
              tunnel: w1769 -> [_ w1789]
              tunnel: w1768 -> [_ w1788]
              tunnel: [w1785 w1786] -> w1767
              frame False {
              }
              frame True {
                n1347 = Subtract(x=w1789, y=w1788) -> (x-y=w1787:i32)
                n1348 = Delete From Array(array=w1791, length=w1787, index=0) -> (array with subset deleted=w1786:dbl[])  [unwired: 1 out]
              }
            }
            "temp buf" <- w1767
          }
        }
      }
      frame Error {
        w1806 = u16 0 items=["None", "XON/XOFF", "RTS/CTS", "XON/XOFF & RTS/CTS", "DTR/DSR", "XON/XOFF & DTR/DSR"] ("flow control (0:none)  2")
        w1804 = u16 10 items=["1.0"=10, "1.5"=15, "2.0"=20] ("stop bits 2")
        w1802 = u16 0 items=["None", "Odd", "Even", "Mark", "Space"] ("parity 2")
        w1803 = u32 10000  # timeout (10sec)
        n1349 = VISA Clear(VISA resource name=w1798, error in (no error)=w1795) -> (VISA resource name out=w1797:refnum<visa-resource-name>, error out=w1796:errorcluster)
        n1350 = VISA Close(VISA resource name=w1797, error in (no error)=w1796) -> (error out=w1799:errorcluster)
        n1351 = call <vilib>:"Clear Errors.vi"("error in (no error)"=w1799) -> ()  [unwired: 5 in, 2 out]
        n1352 = local read "Com Port 2"() -> (w1792:refnum<visa-resource-name>)
        "visa due" <- w1792
        n1353 = call-poly "VISA Configure Serial Port"("VISA resource name"=w1792, "timeout (10sec)"=w1803, "baud rate (9600)"=u32 250000 ("baud rate  2"), "data bits (8)"=u16 8 ("data bits  2"), "parity (0:none)"=w1802, "stop bits (10: 1 bit)"=w1804, "flow control (0:none)"=w1806) -> ("VISA resource name out"=w1807:refnum<visa-resource-name>, "error out"=w1808:errorcluster)  [unwired: 7 in]
        n1354 = flat-sequence {
          tunnel: w1807 -> [w1810]
          tunnel: w1808 -> [w1809]
          tunnel: [w1810] -> w1800
          tunnel: [w1809] -> w1793
          frame #0 {
            n1355 = Wait (ms)(milliseconds to wait=u32 50) -> ()  [unwired: 1 out]
          }
        }
        "Residual Due" <- ""
        "Port 2 Error" <- w1793
      }
    }
    n1356 = local read "Quit"() -> (w1619:bool)
    "Error Due" <- w1627
  }
  n1357 = property on="RUN" class="Bool (strict)"("Visible"=TRUE) -> ()  [unwired: 2 in, 2 out]
  n1358 = while {
    tunnel: [w1828] -> _
    tunnel: [w1812] -> w50
    i -> [w1828]
    stop <- w1812 stop-if-true
    n1359 = local read "conststatus"() -> (w1816:dbl)
    n1360 = local read "Main Tab"() -> (w1814:T2)
    n1361 = local read "EDIT"() -> (w1834:bool)
    n1362 = local read "Rate"() -> (w1833:dbl)
    n1363 = case shown="True" w1834 {
      tunnel: [FALSE TRUE] -> w1820
      frame False {
      }
      frame True {
      }
    }
    n1364 = property on="Time slide" class="Slide (strict)"("Scale.Range:Maximum"=2500.0) -> ()  [unwired: 2 in, 2 out]
    n1365 = Equal?(x=w1814, y=T22."About" ("Main Tab")) -> (x = y?=w1826:bool)
    n1366 = Equal?(x=w1816, y=0.0) -> (x = y?=w1817:bool)
    n1367 = Divide(x=1.0, y=w1833) -> (x/y=w1829:dbl)
    "Time 2" <- w1829
    n1368 = case shown="True" w1817 {
      frame False {
      }
      frame True {
        # "C:\\WinDucom\\calibrate WO 2391.dcf"
        n1369 = local write "Lan flag"(22) -> ()
        n1370 = local write "conststatus"(10.0 ("rpm value : 2")) -> ()
        n1371 = String To Path(string="C:\\LAB-IQ\\calibrate WO 2465.dcf") -> (path=w1840:path)
        n1372 = Open/Create/Replace File "Open File"(file path (use dialog)=w1840) -> (refnum out=w1838:refnum<file>)  [unwired: 5 in, 2 out]
        n1373 = for {
          N: 23 -> [_]
          tunnel: w1838 -> [w1849]
          i -> [w1843]
          (unwired) TRUE ("line mode (F)")
          n1374 = Read from Text File "Read File"(file (use dialog)=w1849) -> (text=w1848:string)  [unwired: 3 in, 3 out]
          n1375 = Match Pattern(string=w1848, regular expression="]") -> (after substring=w1846:string)  [unwired: 1 in, 3 out]
          n1376 = String Subset(string=w1848, offset (0)=5, length (rest)=10 ("length (rest)")) -> (substring=w1841:string)
          n1377 = Fract/Exp String To Number(string=w1841) -> (number=w1842:dbl)  [unwired: 3 in, 1 out]
          n1378 = Match Pattern(string=w1846, regular expression="-") -> (before substring=w1844:string)  [unwired: 1 in, 3 out]
          n1379 = case shown="7" w1843 {
            tunnel: w1842 -> [w1852 w1853 w1854 w1855 _ _ _ w1860 w1861 w1862 w1865 w1866 w1867 w1868 w1869 w1870 w1871 w1874 w1875 _ _ w1878 _ _]
            tunnel: w1844 -> [_ _ _ _ w1856 w1857 w1858 _ _ _ _ _ _ _ _ _ _ _ _ w1876 w1877 _ w1879 _]
            frame 0 {
              n1380 = local write "FRIC. FORCE :"(w1852) -> ()
            }
            frame 1 {
              n1381 = local write "TEMPERATURE :"(w1853) -> ()
            }
            frame 2 {
              n1382 = local write "HUMIDITY:"(w1854) -> ()
            }
            frame 3 {
              n1383 = local write "AIR TEMPERATURE :"(w1855) -> ()
            }
            frame 4 {
              n1384 = local write "Com Port 1"(w1856) -> ()
            }
            frame 5 {
              n1385 = local write "Com Port 2"(w1857) -> ()
              n1386 = local write "visa due"(w1857) -> ()
            }
            frame 6 {
              n1387 = String To Path(string=w1858) -> (path=w1859:path)
              n1388 = local write "File Path"(w1859) -> ()
              "String" <- w1858
            }
            frame 7 {
              n1389 = local write "DISPLACEMENT :"(w1860) -> ()
            }
            frame 8 {
              n1390 = local write "STROKE GAIN :"(w1861) -> ()
            }
            frame 9 {
              n1391 = local read "Stroke PID Gains"() -> (w1864:T8)
              n1392 = Bundle By Name(cluster=w1864, "Proportional Gain (Kc)"=w1862) -> (w1863:T8)
              n1393 = local write "Stroke PID Gains"(w1863) -> ()
            }
            frame 10 {
              n1394 = local write "Language Selection"(w1865) -> ()
            }
            frame 11 {
              n1395 = local write "CH-POWER +"(w1866) -> ()
            }
            frame 12 {
              n1396 = local write "CH-POWER -"(w1867) -> ()
            }
            frame 13 {
              n1397 = local write "CH-HEATER"(w1868) -> ()
            }
            frame 14 {
              n1398 = local write "CH-HUMIDITY WET"(w1869) -> ()
            }
            frame 15 {
              n1399 = local write "CH-HUMIDITY DRY"(w1870) -> ()
            }
            frame 16 {
              n1400 = local read "Stroke PID Gains"() -> (w1873:T8)
              n1401 = Bundle By Name(cluster=w1873, "Integral Time (Ti, min)"=w1871) -> (w1872:T8)
              n1402 = local write "Stroke PID Gains"(w1872) -> ()
            }
            frame 17 {
              n1403 = local write "AIR TEMP INTERCEPT:"(w1874) -> ()
            }
            frame 18 {
              n1404 = local write "TEMP INTERCEPT:"(w1875) -> ()
            }
            frame 19 {
              n1405 = local write "S.NO"(w1876) -> ()
            }
            frame 20 {
              n1406 = local write "Com Port 3"(w1877) -> ()
            }
            frame 21 {
              n1407 = local write "LvdtOff"(w1878) -> ()
            }
            frame 22 {
              n1408 = local write "Humidity :"(w1879) -> ()
            }
            frame 23, Default {
            }
          }
        }
      }
    }
    n1409 = Select(t=u32 2500 ("milliseconds to wait"), s=w1826, f=u32 500 ("milliseconds to wait")) -> (s? t:f=w1824:u32)
    n1410 = Multiply(x=w1829, y=w1824) -> (x*y=w1831:dbl)
    n1411 = property on="FF Calibration g" class="WFGraph (strict)"("Visible"=w1820) -> ()  [unwired: 2 in, 2 out]
    n1412 = property on="Lift" class="Bool (strict)"("Visible"=w1820) -> ()  [unwired: 2 in, 2 out]
    n1413 = property on="Threshold" class="DigNum (strict)"("Visible"=w1820) -> ()  [unwired: 2 in, 2 out]
    n1414 = property on="Time slide" class="Slide (strict)"("Visible"=w1820) -> ()  [unwired: 2 in, 2 out]
    n1415 = call "Elapsed Time2"("Time Target (s)"=w1831, "Auto Reset"=TRUE) -> ("Time has Elapsed"=w1821:bool)  [unwired: 10 in, 7 out]
    n1416 = case shown="True" w1821 {
      frame False {
        # "79.77669138"
        # "2.3554"
        n1417 = local read "FRIC. FORCE :"() -> (w1884:dbl)
        n1418 = local read "FF cal val"() -> (w1881:dbl[])
        n1419 = Multiply(x=w1884, y=79.77669138) -> (x*y=w1883:dbl)
        n1420 = Multiply(x=w1881, y=w1883) -> (x*y=→"FF Calibration g":dbl[])
        "Err Count" <- 0 ("y")
      }
      frame True {
        n1421 = stacked-sequence {
          frame #0 {
            n1422 = stacked-sequence {
              frame #0 {
                "Lift" <- TRUE ("Lift")
              }
            }
          }
          frame #1 {
            w1896 = 2500 ("y")
            n1423 = local read "RUN"() -> (w1888:bool)
            n1424 = local read "FF1"() -> (w1891:dbl[])
            n1425 = case shown="False" w1888 {
              frame False {
                n1426 = local write "Frequency"(0.0 ("Frequency")) -> ()
              }
              frame True {
              }
            }
            n1427 = Array Size(array=w1891) -> (size(s)=w1890:i32)
            n1428 = local read "Ch1"() -> (w1887:dbl[])
            "Waveform Chart 2" <- w1887
            n1429 = call-poly <vilib>:"Mean.vi"("X"=w1887) -> ("mean"=→"Raw Mean":dbl)  [unwired: 1 out]
            n1430 = Insert Into Array(array=w1891, index=w1890, new element=w1887) -> (w1893:dbl[])
            n1431 = Array Size(array=w1893) -> (size(s)=w1897:i32)
            n1432 = Subtract(x=w1897, y=w1896) -> (x-y=w1895:i32)
            n1433 = Greater?(x=w1897, y=w1896) -> (0:w1898:bool)
            n1434 = case shown="True" w1898 {
              tunnel: w1895 -> [_ w1902]
              tunnel: [w1900 w1904] -> w1889
              tunnel: w1893 -> [w1900 w1903]
              frame False {
              }
              frame True {
                n1435 = Delete From Array(array=w1903, length=w1902, index=0) -> (array with subset deleted=w1904:dbl[])  [unwired: 1 out]
                "Numeric" <- w1902
              }
            }
            "FF1" <- w1889
            "PID Ref" <- TRUE ("PID Ref")
          }
          frame #2 {
          }
          frame #3 {
            # "CONVERT TO N"
            # "DATA PROCESSING"
            # "115 mV/N"
            n1436 = local read "RH Numeric:"() -> (w1909:dbl)
            n1437 = local read "HUMIDITY:"() -> (w1910:dbl)
            n1438 = local read "temp buf"() -> (w1971:dbl[])
            n1439 = local read "Air temp"() -> (w1969:dbl[])
            n1440 = local read "ecr buf"() -> (w1931:dbl[])
            n1441 = local read "Fric Val"() -> (w1975:dbl[])
            n1442 = case shown="True" "Boolean 5" {
              frame False {
              }
              frame True {
                n1443 = local write "Boolean 5"(FALSE) -> ()
                n1444 = local write "Captured Values"(dbl[][] [] ("Captured Values")) -> ()
                n1445 = local write "Best Fit"(dbl[] [] ("Best Fit")) -> ()
              }
            }
            n1446 = local read "TEMPERATURE :"() -> (w1952:dbl)
            n1447 = call-poly <vilib>:"Mean.vi"("X"=w1931) -> ("mean"=w1928:dbl)  [unwired: 1 out]
            n1448 = call-poly <vilib>:"Mean.vi"("X"=w1969) -> ("mean"=w1938:dbl)  [unwired: 1 out]
            "Raw air temp" <- w1938
            n1449 = call-poly <vilib>:"Mean.vi"("X"=w1971) -> ("mean"=w1940:dbl)  [unwired: 1 out]
            "Raw specimen temp" <- w1940
            n1450 = local read "TEMP INTERCEPT:"() -> (w1945:dbl)
            n1451 = Multiply(x=w1909, y=w1910) -> (x*y=→"Humidity ( %RH )" →"Hum" →"Hum 2":dbl)
            n1452 = Multiply(x=w1975, y=1.0) -> (x*y=w1976:dbl[])
            n1453 = local read "FRIC. FORCE :"() -> (w1968:dbl)
            n1454 = Multiply(x=w1940, y=w1952) -> (x*y=w1934:dbl)
            n1455 = local read "AIR TEMPERATURE :"() -> (w1953:dbl)
            n1456 = local read "RUN"() -> (w1965:bool)
            n1457 = Add(x=w1938, y="Offset Air Temp") -> (x+y=w1933:dbl)
            n1458 = local read "AIR TEMP INTERCEPT:"() -> (w1949:dbl)
            n1459 = case shown="0, Default" "Calibrating" {
              tunnel: w1940 -> [w1995 _]
              tunnel: [w1995 w1996] -> w1939
              tunnel: w1938 -> [_ w1996]
              frame 0, Default {
              }
              frame 1 {
              }
            }
            n1460 = Multiply(x=w1928, y="ECR_Gain") -> (x*y=w1927:dbl)
            n1461 = Add(x=w1934, y=w1945) -> (x+y=w1950:dbl)
            n1462 = Multiply(x=w1968, y=79.77669138) -> (x*y=w1966:dbl)
            n1463 = Select(t=0.01 ("FF fil1"), s=w1965, f=0.1 ("FF fil1")) -> (s? t:f=w1961:dbl)
            n1464 = local read "ecr"() -> (w1922:dbl)
            n1465 = Multiply(x=w1933, y=w1953) -> (x*y=w1935:dbl)
            n1466 = Multiply(x=w1976, y=w1966) -> (x*y=w1973:dbl[])
            n1467 = Multiply(x=w1927, y=0.2) -> (x*y=w1920:dbl)
            n1468 = Multiply(x=0.8, y=w1922) -> (x*y=w1921:dbl)
            n1469 = call <vilib>:"Mean PtByPt.vi"("x"=w1950, "sample length"=10) -> ("mean"=w1911:dbl)  [unwired: 2 in, 1 out]
            "TEMP 2" <- w1911
            "TEMP 3" <- w1911
            n1470 = local read "AIR TEMP"() -> (w1958:dbl)
            n1471 = Add(x=w1935, y=w1949) -> (x+y=w1951:dbl)
            n1472 = call-poly <vilib>:"Mean.vi"("X"=w1973) -> ("mean"=w1974:dbl)  [unwired: 1 out]
            n1473 = Add(x=w1920, y=w1921) -> (x+y=w1919:dbl)
            n1474 = Subtract(x=1.0 ("y"), y=w1961) -> (x-y=w1959:dbl)
            n1475 = local write "TEMP"(w1911) -> ()
            n1476 = Multiply(x=w1959, y=w1958) -> (x*y=w1957:dbl)
            n1477 = Multiply(x=w1951, y=w1961) -> (x*y=w1962:dbl)
            n1478 = Not A Number/Path/Refnum?(number/path/refnum=w1919) -> (NaN/Path/Refnum?=w1929:bool)
            n1479 = Subtract(x=w1973, y=w1974) -> (x-y=w1944:dbl[])
            n1480 = local read "FRICVALZ"() -> (w1983:dbl)
            n1481 = case shown="True" "Boolean 4" {
              tunnel: w1939 -> [_ w2002]
              tunnel: "Standard Temp. ( °c )" -> [_ w2001]
              frame False {
              }
              frame True {
                n1482 = Build Array(w2001, w2002) -> (w2000:dbl[])
                n1483 = local write "Boolean 4"(FALSE ("Boolean 4")) -> ()
                n1484 = local read "Captured Values"() -> (w1999:dbl[][])
                n1485 = Build Array (concatenate)(w1999, w2000) -> (w1997:dbl[][])
                n1486 = local write "Captured Values"(w1997) -> ()
              }
            }
            n1487 = Compound Arithmetic op=OR("FRICVALZ 4", "FRICVALZ 3", "FRICVALZ 2") -> (w1913:bool)
            n1488 = Add(x=w1962, y=w1957) -> (x+y=w1955:dbl)
            n1489 = Absolute Value(x=w1944) -> (abs(x)=w1978:dbl[])
            n1490 = call-poly <vilib>:"RMS.vi"("X"=w1944) -> ("rms value"=w1943:dbl)  [unwired: 1 out]
            n1491 = Select(t=0.0, s=w1929, f=w1919) -> (s? t:f=w1926:dbl)
            n1492 = call-poly <vilib>:"Mean.vi"("X"=w1978) -> ()  [unwired: 2 out]
            n1493 = local read "FF 2"() -> (w1985:dbl)
            n1494 = case shown="True" w1913 {
              tunnel: w1943 -> [_ w2007]
              frame False {
              }
              frame True {
                w2006 = FALSE ("FRICVALZ")
                n1495 = local write "FRICVALZ 3"(w2006) -> ()
                n1496 = local write "FRICVALZ 2"(w2006) -> ()
                n1497 = local write "FRICVALZ 4"(w2006) -> ()
                "FRICVALZ" <- w2007
              }
            }
            n1498 = Subtract(x=w1943, y=w1983) -> (x-y=w1977:dbl)
            n1499 = Not A Number/Path/Refnum?(number/path/refnum=w1955) -> (NaN/Path/Refnum?=w1956:bool)
            n1500 = In Range and Coerce(upper limit=100.0, x=w1926, lower limit=0.0) -> ()  [unwired: 2 out]
            n1501 = Select(t=0.0, s=w1956, f=w1955) -> (s? t:f=w1916:dbl)
            "AIR TEMP" <- w1916
            n1502 = Multiply(x=w1977, y=0.1 ("FF fil1")) -> (x*y=w1989:dbl)
            n1503 = Multiply(x=0.9 ("FF fil2"), y=w1985) -> (x*y=w1988:dbl)
            n1504 = call "Elapsed Time11"("Time Target (s)"=1.0) -> ("Time has Elapsed"=w1918:bool)  [unwired: 11 in, 7 out]
            n1505 = Add(x=w1989, y=w1988) -> (x+y=w1906:dbl)
            "FF 2" <- w1906
            "FF 4" <- w1906
            n1506 = local read "NORMAL LOAD"() -> (w1972:dbl)
            n1507 = case shown="True" w1918 {
              tunnel: w1916 -> [_ w1991]
              frame False {
              }
              frame True {
                "AirT" <- w1991
              }
            }
            n1508 = local read "TEMP"() -> (w1982:dbl)
            n1509 = local write "FF 3"(w1906) -> ()
            n1510 = Not A Number/Path/Refnum?(number/path/refnum=w1906) -> (NaN/Path/Refnum?=w1980:bool)
            n1511 = Divide(x=w1906, y=w1972) -> (x/y=w1946:dbl)
            n1512 = Not A Number/Path/Refnum?(number/path/refnum=w1982) -> (NaN/Path/Refnum?=w1981:bool)
            n1513 = Compound Arithmetic op=OR(w1981, w1980) -> (w1979:bool)
            n1514 = Not A Number/Path/Refnum?(number/path/refnum=w1946) -> (NaN/Path/Refnum?=w1947:bool)
            n1515 = case shown="True" w1979 {
              frame False {
              }
              frame True {
                n1516 = local write "TEMP"(0.0 ("TEMP")) -> ()
                n1517 = local write "FF 2"(0.0 ("FF 2")) -> ()
                n1518 = local write "reinit"(TRUE ("reinit")) -> ()
              }
            }
            n1519 = Select(t=0.0, s=w1947, f=w1946) -> (s? t:f=w1907:dbl)
            "COF 2" <- w1907
            n1520 = local write "COF 3"(w1907) -> ()
          }
          frame #4 {
            n1521 = flat-sequence {
              frame #0 {
                n1522 = Wait (ms)(milliseconds to wait=u32 100) -> ()  [unwired: 1 out]
              }
              frame #1 {
                n1523 = local write "Lift"(FALSE ("Lift")) -> ()
              }
            }
            n1524 = case shown="True" "Boolean 6" {
              frame False {
              }
              frame True {
                n1525 = local write "Boolean 6"(FALSE ("Boolean 6")) -> ()
                n1526 = local read "Captured Values"() -> (w2018:dbl[][])
                n1527 = Index Array(array=w2018, index (col) #1=0 ("disabled index (col)"), index (col) #2=1 ("index (col)")) -> (element #1=w2016:dbl[], element #2=w2014:dbl[])  [unwired: 2 in]
                n1528 = call <vilib>:"Linear Fit.vi"("Y"=w2016, "X"=w2014) -> ("Best Linear Fit"=→"Best Fit":dbl[], "slope"=w2010:dbl, "intercept"=w2009:dbl)  [unwired: 9 in, 2 out]
                "Slope" <- w2010
                "Intercept" <- w2009
                n1529 = local read "Calibrating"() -> (w2011:u16)
                n1530 = case shown="1" w2011 {
                  tunnel: w2010 -> [w2020 w2022]
                  tunnel: w2009 -> [w2019 w2021]
                  frame 0, Default {
                    n1531 = local write "TEMPERATURE :"(w2020) -> ()
                    n1532 = local write "TEMP INTERCEPT:"(w2019) -> ()
                  }
                  frame 1 {
                    n1533 = local write "AIR TEMPERATURE :"(w2022) -> ()
                    n1534 = local write "AIR TEMP INTERCEPT:"(w2021) -> ()
                  }
                }
              }
            }
          }
        }
      }
    }
    n1535 = Wait (ms)(milliseconds to wait=u32 50) -> ()  [unwired: 1 out]
    n1536 = local read "Quit"() -> (w1812:bool)
    "Rate" <- 2500.0 ("No of Samples")
    "Humid Last buf" <- dbl[] [0.0, 0.0, 0.0, 0.0] ("Humid Last buf")
  }
  n1537 = while {
    tunnel: w55 -> [_]
    tunnel: [w2052] -> _
    tunnel: [w2027] -> w52
    i -> [w2052]
    stop <- w2027 stop-if-true
    # "C:\\LAB-IQ-NXT\\Scar View.exe"
    n1538 = local read "OK Button 16"() -> (w2041:bool)
    n1539 = local read "Re-Initialise"() -> (w2037:bool)
    n1540 = local read "Main Tab"() -> (w2033:T2)
    n1541 = local read "service 3"() -> (w2034:bool)
    n1542 = local read "OPEN 6"() -> (w2036:bool)
    n1543 = local read "EDIT 2"() -> (w2039:bool)
    n1544 = flat-sequence {
      frame #0 {
        n1545 = stacked-sequence {
          frame #0 {
            n1546 = local read "EDIT"() -> (w2707:bool)
            n1547 = case shown="True" w2707 {
              tunnel: [u8 2 ("Disabled") u8 0 ("Disabled")] -> _
              frame False {
                w2709 = FALSE
                n1548 = local write "Password"("") -> ()
                n1549 = property on="SrvM CP" class="Bool (strict)"("Visible"=w2709) -> ()  [unwired: 2 in, 2 out]
                n1550 = property on="message" class="Str"("Visible"=w2709) -> ()  [unwired: 2 in, 2 out]
                n1551 = local write "x = y?"(w2709) -> ()
                n1552 = property on="Password" class="Str"("Visible"=w2709) -> ()  [unwired: 2 in, 2 out]
                n1553 = property on="ENTER THE NEW PASSWORD" class="Str"("Visible"=w2709) -> ()  [unwired: 2 in, 2 out]
                n1554 = property on="ENTER CURRENT PASSWORD" class="Str"("Visible"=w2709) -> ()  [unwired: 2 in, 2 out]
                n1555 = local write "SrvM CP"(w2709) -> ()
              }
              frame True {
                w2712 = TRUE
                n1556 = property on="SrvM CP" class="Bool (strict)"("Visible"=w2712) -> ()  [unwired: 2 in, 2 out]
                n1557 = property on="Password" class="Str"("Visible"=w2712) -> ()  [unwired: 2 in, 2 out]
              }
            }
            "dipl pwd" <- "@143$\n" ("dipl pwd")
          }
          frame #1 {
            # "Gain password"
            n1558 = String To Byte Array(string="ENTER CURRENT PASSWORD") -> (unsigned byte array=w2717:u8[])
            n1559 = Search 1D Array(1D array=w2717, element=u8 10) -> (index of element=w2720:i32)  [unwired: 1 in]
            n1560 = Index Array(array=w2717, index=w2720) -> (element=w2716:u8)
            n1561 = Equal?(x=w2716, y=10) -> (x = y?=w2714:bool)
            n1562 = case shown="True" w2714 {
              frame False {
                n1563 = property on="ENTER THE NEW PASSWORD" class="Str"("Visible"=FALSE) -> ()  [unwired: 2 in, 2 out]
              }
              frame True {
